vi "Periodic Tasks.vi"(7 "Chassis X SPD":dbl=0.7, 8 "error in":errorcluster) -> ()   [LabVIEW 2019]
doc: "This VI runs in parallel to other tasks. It can contain as many user-defined periodic loops as you need. These can carry out PID or other sorts of timed response."
uses:
  <vilib>/Rock Robotics/WPI/Utilities/WPI_GetSetVariantRefNum.vi
  Robot Global Data.vi
  <vilib>/Rock Robotics/Network Tables/NT Write Number.vi
  <vilib>/Rock Robotics/Network Tables/NT Read Number.vi
  <vilib>/Rock Robotics/Network Tables/NT Read Boolean.vi
  <vilib>/Rock Robotics/WPI/RobotDrive/WPI_RobotDriveArcadeDrive_Standard(NoSaturation).vi
panel:
  in  "Chassis Y SPD":dbl=0.7
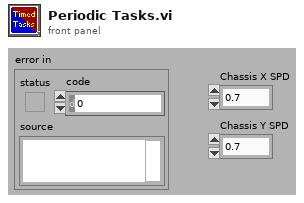
[diagram p1: front panel]
types:
  T1 = typedef "WPI_JoystickDevRef.ctl" = cluster{"Device":T2}
  T2 = typedef "WPI_JoystickDeviceEnum.ctl" = enum16{"USB 0", "USB 1", "USB 2", "USB 3", "USB 4", "USB 5"}
  T3 = typedef "WPI_RobotDriveDevRef.ctl" = cluster{"DevStatus":errorcluster, "Motors[]":T4[], "Square Inputs":bool, "Max Output":dbl}
  T4 = typedef "WPI_MotorControlDeviceRef.ctl" = cluster{"DeviceStatus":errorcluster, "Type":T5, "PWM":cluster{"PWM Channel":T6, "DeadBand":T7}, "CAN":cluster{"Device Number":u8, "SetOutput VI Ref":variant, "GetOutput VI Ref":variant, "Enable VI Ref":variant, "Disable VI Ref":variant, "Data":variant}, "Invert":bool, "DIO PWM":cluster{"PWM \"Enable\" Channel":T6, "DIOChannel":T8, "PWM Rate":dbl}}
  T5 = typedef "WPI_MotorControlType.ctl" = enum16{"PWM", "CAN", "DIO PWM"}
  T6 = typedef "FPGA_DIOPWMChannel.ctl" = enum8{"PWM 0", "PWM 1", "PWM 2", "PWM 3", "PWM 4", "PWM 5", "PWM 6", "PWM 7", "PWM 8", "PWM 9", "PWM MXP 0", "PWM MXP 1", "PWM MXP 2", "PWM MXP 3", "PWM MXP 4", "PWM MXP 5", "PWM MXP 6", "PWM MXP 7", "PWM MXP 8", "PWM MXP 9", "Invalid"}
  T7 = typedef "WPI_PWMDeadband.ctl" = cluster{"Name":string, "maxPositivePwm":i32, "minPositivePwm":i32, "centerPwm":i32, "maxNegativePwm":i32, "minNegativePwm":i32, "angularRange":u16}
  T8 = typedef "FPGA_DIOChannel.ctl" = enum8{"DIO 0", "DIO 1", "DIO 2", "DIO 3", "DIO 4", "DIO 5", "DIO 6", "DIO 7", "DIO 8", "DIO 9", "DIO MXP 0", "DIO MXP 1", "DIO MXP 2", "DIO MXP 3", "DIO MXP 4", "DIO MXP 5", "DIO MXP 6", "DIO MXP 7", "DIO MXP 8", "DIO MXP 9", "DIO MXP 10", "DIO MXP 11", "DIO MXP 12", "DIO MXP 13", "DIO MXP 14", "DIO MXP 15", "SPI Port CS1", "SPI Port CS2", "SPI Port CS3", "SPI Port MISO", "SPI Port MOSI", "Invalid"}
  T9 = cluster{"JoystickDevRef":T1, "RobotDriveDevRef":T3}
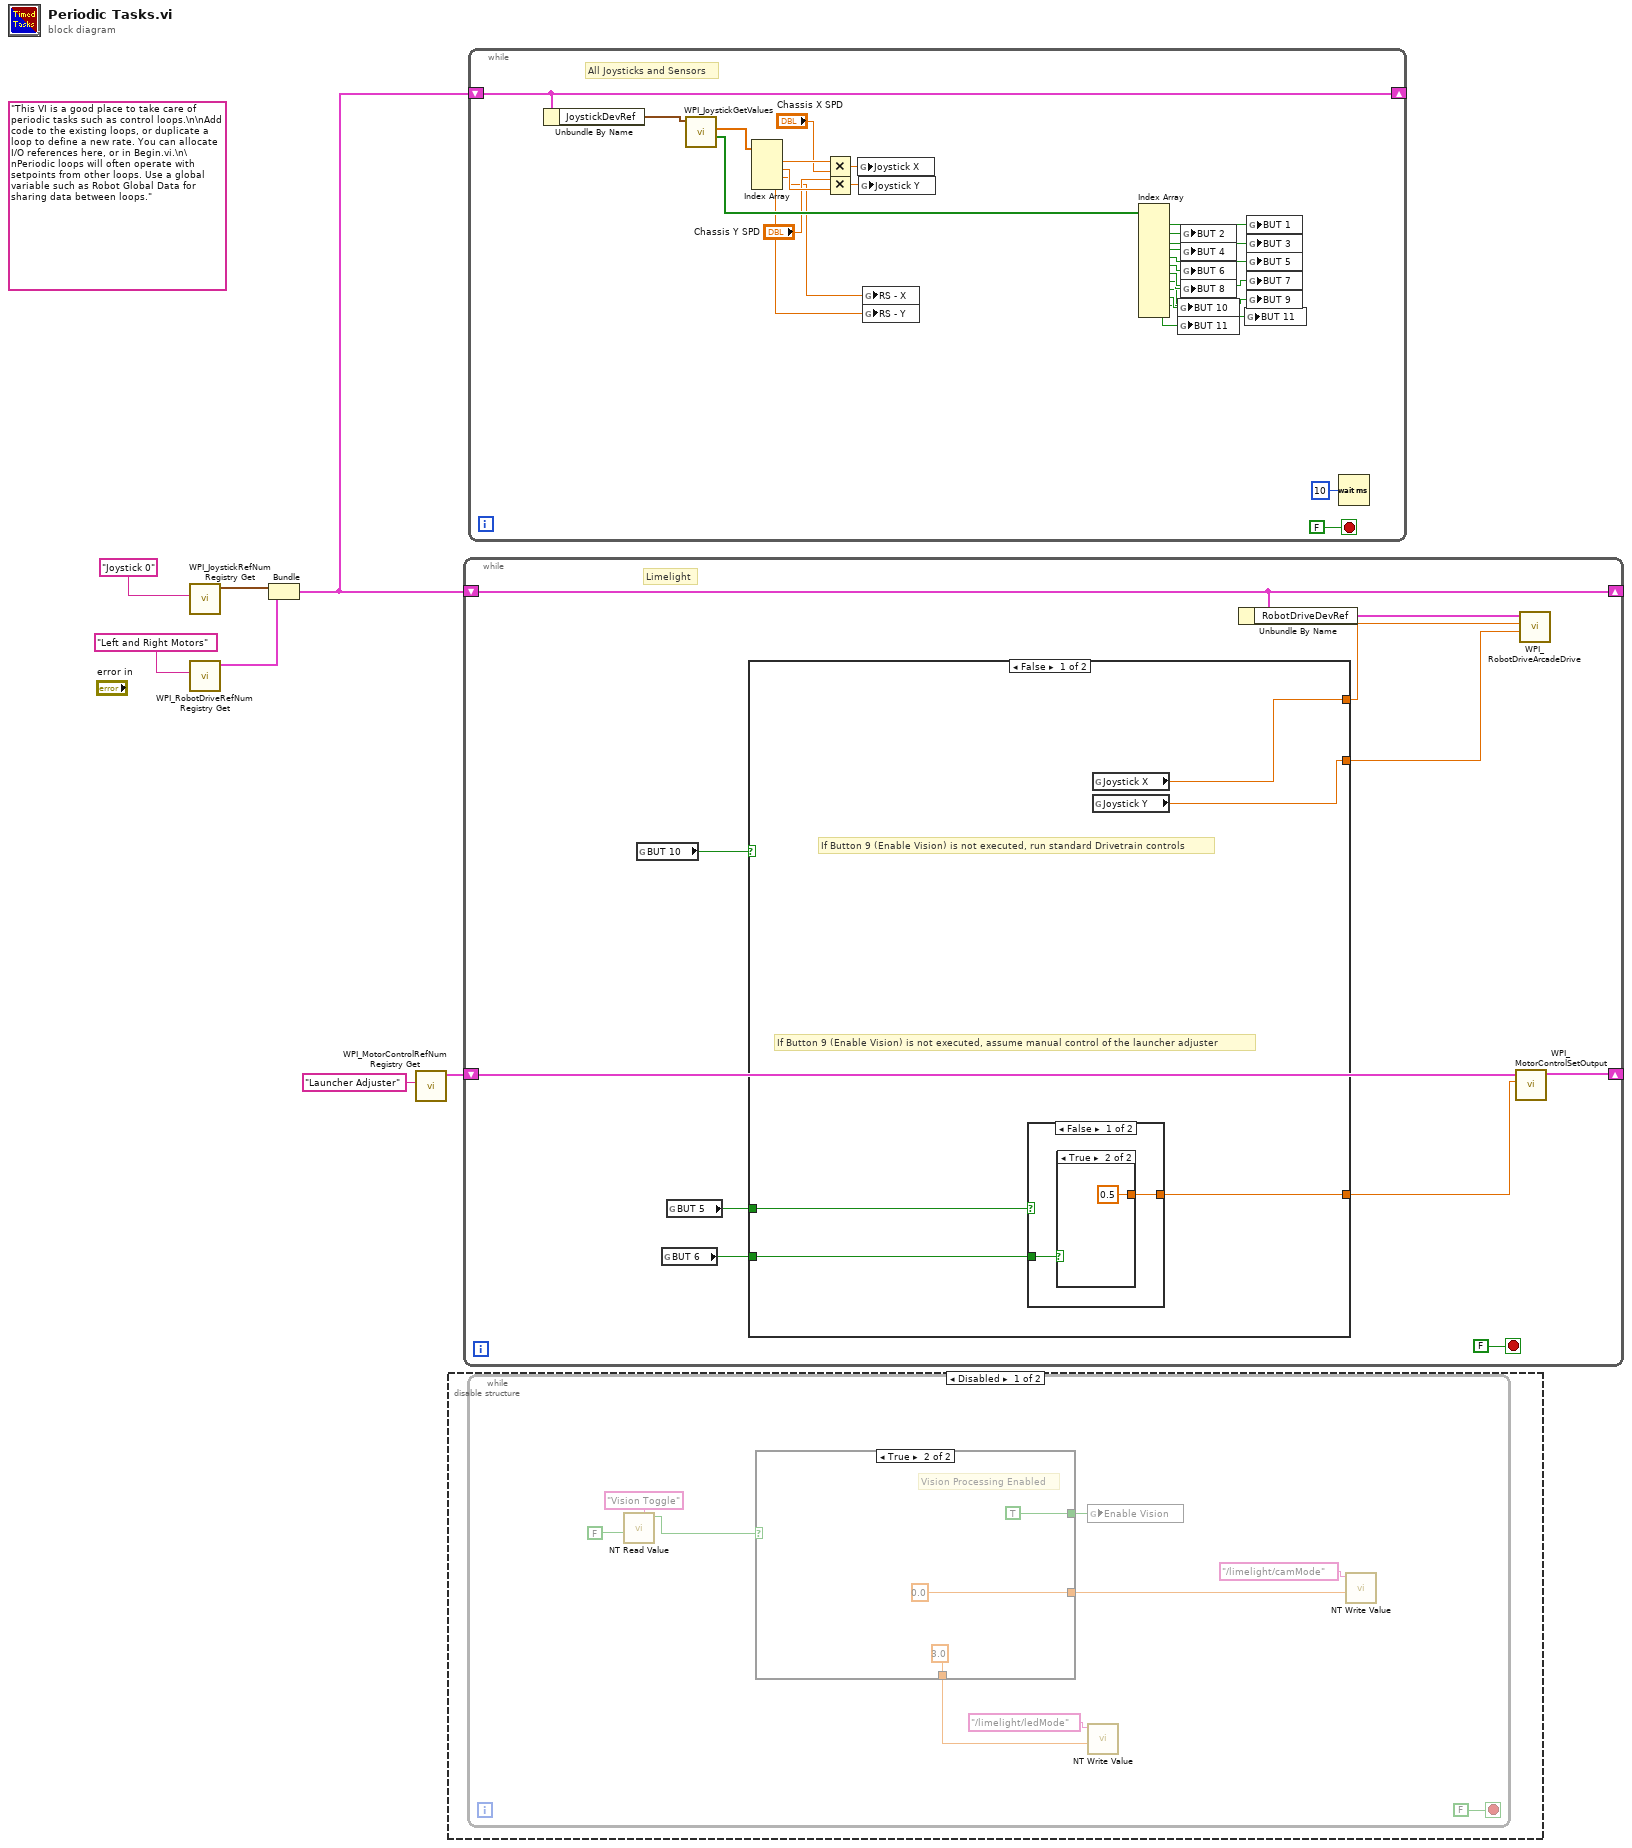
[diagram p0: block diagram]
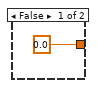
[diagram p2: hidden frame]
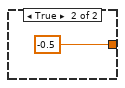
[diagram p3: hidden frame]
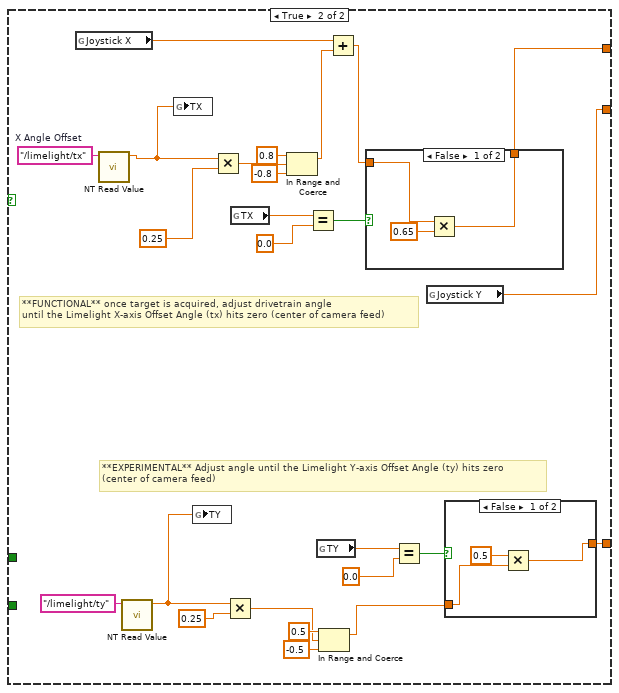
[diagram p4: hidden frame]
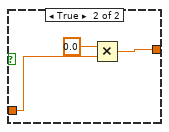
[diagram p5: hidden frame]
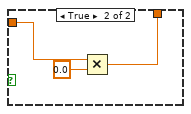
[diagram p6: hidden frame]
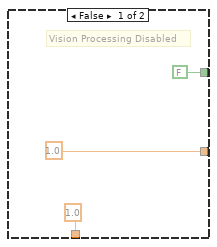
[diagram p7: hidden frame]
diagram:
  (unwired) "This VI is a good place to take care of periodic tasks such as control loops.\n\nAdd code to the existing loops, or duplicate a loop to define a new rate. You can allocate I/O references here, or in Begin.vi.\n\nPeriodic loops will often operate with setpoints from other loops. Use a global variable such as Robot Global Data for sharing data between loops."
  n1 = call <vilib>:"WPI_JoystickRefNum Registry Get.vi"("refnum name"="Joystick 0") -> ("JoystickDevRef"=w5:T1)  [unwired: 1 in, 9 out]
  n2 = call <vilib>:"WPI_RobotDriveRefNum Registry Get.vi"("refnum name"="Left and Right Motors") -> ("RobotDriveDevRef"=w4:T3)  [unwired: 1 in, 9 out]
  n3 = Bundle("JoystickDevRef"=w5, "RobotDriveDevRef"=w4) -> (w3:T9)  [unwired: 1 out]
  n4 = call <vilib>:"WPI_MotorControlRefNum Registry Get.vi"("refnum name"="Launcher Adjuster") -> ("MotorControlDevRef"=w2:T4)  [unwired: 9 in, 1 out]
  n5 = disable-structure shown="Disabled" {
    frame Disabled {
      n6 = while {
        stop <- FALSE stop-if-true
        n7 = call-poly <vilib>:"NT Read Value.vi"("Default Value"=FALSE, "Name"="Vision Toggle") -> ("Boolean"=w16:bool)  [unwired: 8 in, 1 out]
        n8 = case shown="True" w16 {
          tunnel: [FALSE ("Enable Vision") TRUE ("Enable Vision")] -> w13
          tunnel: [1.0 ("Numeric") 0.0 ("Numeric")] -> w14
          tunnel: [1.0 ("Numeric") 3.0 ("Numeric")] -> w15
          frame False {
            # "Vision Processing Disabled"
          }
          frame True {
            # "Vision Processing Enabled"
          }
        }
        n9 = global write "Robot Global Data.vi" "Enable Vision"(w13) -> ()
        n10 = call-poly <vilib>:"NT Write Value.vi"("Numeric"=w15, "Name"="/limelight/ledMode") -> ()  [unwired: 9 in, 1 out]
        n11 = call-poly <vilib>:"NT Write Value.vi"("Numeric"=w14, "Name"="/limelight/camMode") -> ()  [unwired: 9 in, 1 out]
      }
    }
    frame Enabled {
    }
  }
  n12 = while {
    shift-right: [w32] -> _
    shift-left: w3 -> [w32]
    shift-right: [w27] -> _
    shift-left: w2 -> [w26]
    stop <- FALSE stop-if-true
    # "Limelight"
    n13 = global read "Robot Global Data.vi" "BUT 10"() -> (w31:bool)
    n14 = global read "Robot Global Data.vi" "BUT 6"() -> (w23:bool)
    n15 = global read "Robot Global Data.vi" "BUT 5"() -> (w24:bool)
    n16 = case shown="False" w31 {
      tunnel: [w38 w59] -> w29
      tunnel: [w37 w55] -> w28
      tunnel: [w36 w48] -> w25
      tunnel: w24 -> [w35 _]
      tunnel: w23 -> [w34 _]
      frame False {
        # "If Button 9 (Enable Vision) is not executed, assume manual control of the launcher adjuster"
        # "If Button 9 (Enable Vision) is not executed, run standard Drivetrain controls"
        n17 = case shown="False" w35 {
          tunnel: [w40 -0.5] -> w36
          tunnel: w34 -> [w39 _]
          frame False {
            n18 = case shown="True" w39 {
              tunnel: [0.0 0.5] -> w40
              frame False {
              }
              frame True {
              }
            }
          }
          frame True {
          }
        }
        n19 = global read "Robot Global Data.vi" "Joystick X"() -> (w38:dbl)
        n20 = global read "Robot Global Data.vi" "Joystick Y"() -> (w37:dbl)
      }
      frame True {
        w68 = "/limelight/tx"  # X Angle Offset
        # "**FUNCTIONAL** once target is acquired, adjust drivetrain angle \nuntil the Limelight X-axis Offset Angle (tx) hits zero (center of camera feed)"
        # "**EXPERIMENTAL** Adjust angle until the Limelight Y-axis Offset Angle (ty) hits zero\n(center of camera feed)"
        n21 = global read "Robot Global Data.vi" "Joystick X"() -> (w67:dbl)
        n22 = call-poly <vilib>:"NT Read Value.vi"("Name"=w68) -> ("Numeric"=w61:dbl)  [unwired: 9 in, 1 out]
        n23 = call-poly <vilib>:"NT Read Value.vi"("Name"="/limelight/ty") -> ("Numeric"=w53:dbl)  [unwired: 9 in, 1 out]
        n24 = global write "Robot Global Data.vi" "TX"(w61) -> ()
        n25 = global write "Robot Global Data.vi" "TY"(w53) -> ()
        n26 = Multiply(x=w61, y=0.25) -> (x*y=w65:dbl)
        n27 = Multiply(x=w53, y=0.25) -> (x*y=w45:dbl)
        n28 = global read "Robot Global Data.vi" "TX"() -> (w57:dbl)
        n29 = In Range and Coerce(upper limit=0.8, x=w65, lower limit=-0.8) -> (coerced(x)=w66:dbl)  [unwired: 1 out]
        n30 = Equal?(x=w57, y=0.0) -> (x = y?=w58:bool)
        n31 = global read "Robot Global Data.vi" "TY"() -> (w51:dbl)
        n32 = In Range and Coerce(upper limit=0.5, x=w45, lower limit=-0.5) -> (coerced(x)=w44:dbl)  [unwired: 1 out]
        n33 = Add(x=w67, y=w66) -> (x+y=w60:dbl)
        n34 = case shown="False" w58 {
          tunnel: w60 -> [w76 w80]
          tunnel: [w77 w78] -> w59
          frame False {
            n35 = Multiply(x=w76, y=0.65) -> (x*y=w77:dbl)
          }
          frame True {
            n36 = Multiply(x=w80, y=0.0) -> (x*y=w78:dbl)
          }
        }
        n37 = Equal?(x=w51, y=0.0) -> (x = y?=w49:bool)
        n38 = global read "Robot Global Data.vi" "Joystick Y"() -> (w55:dbl)
        n39 = case shown="False" w49 {
          tunnel: [w69 w74] -> w48
          tunnel: w44 -> [w71 w73]
          frame False {
            n40 = Multiply(x=0.5, y=w71) -> (x*y=w69:dbl)
          }
          frame True {
            n41 = Multiply(x=0.0, y=w73) -> (x*y=w74:dbl)
          }
        }
      }
    }
    n42 = Unbundle By Name(w32) -> ("RobotDriveDevRef"=w30:T3)
    n43 = call <vilib>:"WPI_MotorControlSetOutput.vi"("Output"=w25, "MotorControlDevRef"=w26) -> ("MotorControlDevRef"=w27:T4)  [unwired: 7 in, 2 out]
    n44 = call-poly <vilib>:"WPI_RobotDriveArcadeDrive.vi"("Y axis value"=w28, "X axis value"=w29, "RobotDriveDevRef"=w30) -> ()  [unwired: 6 in, 3 out]
  }
  n45 = while {
    shift-right: [w90] -> _
    shift-left: w3 -> [w90]
    stop <- FALSE stop-if-true
    # "All Joysticks and Sensors"
    n46 = Unbundle By Name(w90) -> ("JoystickDevRef"=w104:T1)
    n47 = call <vilib>:"WPI_JoystickGetValues.vi"("JoystickDevRef"=w104) -> ("Buttons"=w103:bool[], "Axes"=w89:dbl[])  [unwired: 6 in, 3 out]
    n48 = Index Array(array=w89) -> (element #1=w86:dbl, element #2=w85:dbl, element #3=w82:dbl, element #4=w81:dbl)  [unwired: 4 in]
    n49 = Multiply(x=w86, y="Chassis X SPD") -> (x*y=w88:dbl)
    n50 = Multiply(x="Chassis Y SPD", y=w85) -> (x*y=w87:dbl)
    n51 = global write "Robot Global Data.vi" "Joystick X"(w88) -> ()
    n52 = global write "Robot Global Data.vi" "Joystick Y"(w87) -> ()
    n53 = global write "Robot Global Data.vi" "RS - X"(w82) -> ()
    n54 = global write "Robot Global Data.vi" "RS - Y"(w81) -> ()
    n55 = Index Array(array=w103) -> (element #1=w102:bool, element #2=w101:bool, element #3=w100:bool, element #4=w99:bool, element #5=w98:bool, element #6=w97:bool, element #7=w96:bool, element #8=w95:bool, element #9=w94:bool, element #10=w93:bool, element #11=w92:bool, element #12=w91:bool)  [unwired: 12 in]
    n56 = global write "Robot Global Data.vi" "BUT 10"(w93) -> ()
    n57 = global write "Robot Global Data.vi" "BUT 11"(w91) -> ()
    n58 = global write "Robot Global Data.vi" "BUT 2"(w101) -> ()
    n59 = global write "Robot Global Data.vi" "BUT 4"(w99) -> ()
    n60 = global write "Robot Global Data.vi" "BUT 6"(w97) -> ()
    n61 = global write "Robot Global Data.vi" "BUT 8"(w95) -> ()
    n62 = global write "Robot Global Data.vi" "BUT 11"(w92) -> ()
    n63 = global write "Robot Global Data.vi" "BUT 1"(w102) -> ()
    n64 = global write "Robot Global Data.vi" "BUT 3"(w100) -> ()
    n65 = global write "Robot Global Data.vi" "BUT 5"(w98) -> ()
    n66 = global write "Robot Global Data.vi" "BUT 7"(w96) -> ()
    n67 = global write "Robot Global Data.vi" "BUT 9"(w94) -> ()
    n68 = Wait (ms)(milliseconds to wait=u32 10) -> ()  [unwired: 1 out]
  }
